vi "Switching Passive Active, Waveform Parameters.vi"(0 "error in":errorcluster, 3 "waveform":i32=1 min=1 step=1) -> (7 "error out":errorcluster, 10 "MICS Command":string)   [LabVIEW 2010]
doc: "This function builds the Patient Stim programs for Switching Passive Active."
panel:
  in  "Patient Stim Program":string[][](table)=[["ProgramNumber", "4", "4"], ["ProgramDefined", "1", "1"], ["ProgramDisabled", "0", "0"], ["ProgramName", "4_P-A Switch_3x8", "4_P-A Switch_2x12"], ["AllowedFrequencies[0]", "0xFF", "0xFF"], ["AllowedFrequencies[1]", "0xFF", "0xFF"], ["AllowedFrequencies[2]", "0xFF", "0xFF"], ["AllowedFrequencies[3]", "0xFF", "0xFF"], ["AllowedFrequencies[4]", "0xFF", "0xFF"], ["AllowedFrequencies[5]", "0xFF", "0xFF"], ["AllowedFrequencies[6]", "0xFF", "0xFF"], ["AllowedFrequencies[7]", "0xFF", "0xFF"], ["ProgramFrequencyIndex", "21", "21"], ["DefinedPulseMap", "15", "15"], ["PulseNamePA", "P1", "P1"], ["AmplitudeLowLimitPA", "5000", "5000"], ["AmplitudeStepPA", "15", "15"], ["AmplitudeStepIndexPA", "1", "1"], ["PulseWidthLowLimitPA", "400", "400"], ["PulseWidthHighLimitPA", "600", "600"], ["PulseWidthPA", "500", "500"], ["ElectrodeAmpPercentagePA[CH01]", "0", "0"], ["ElectrodeAmpPercentagePA[CH02]", "0", "0"], ["ElectrodeAmpPercentagePA[CH03]", "0", "0"], ["ElectrodeAmpPercentagePA[CH04]", "0", "0"], ["ElectrodeAmpPercentagePA[CH05]", "0", "0"], ["ElectrodeAmpPercentagePA[CH06]", "0", "0"], ["ElectrodeAmpPercentagePA[CH07]", "0", "0"], ["ElectrodeAmpPercentagePA[CH08]", "0", "0"], ["ElectrodeAmpPercentagePA[CH09]", "0", "0"], ["ElectrodeAmpPercentagePA[CH10]", "0", "0"], ["ElectrodeAmpPercentagePA[CH11]", "0", "0"], ["ElectrodeAmpPercentagePA[CH12]", "0", "0"], ["ElectrodeAmpPercentagePA[CH13]", "0", "0"], ["ElectrodeAmpPercentagePA[CH14]", "0", "0"], ["ElectrodeAmpPercentagePA[CH15]", "0", "0"], ["ElectrodeAmpPercentagePA[CH16]", "100", "0"], ["ElectrodeAmpPercentagePA[CH17]", "-100", "100"], ["ElectrodeAmpPercentagePA[CH18]", "0", "0"], ["ElectrodeAmpPercentagePA[CH19]", "0", "-100"], ["ElectrodeAmpPercentagePA[CH20]", "0", "0"], ["ElectrodeAmpPercentagePA[CH21]", "0", "0"], ["ElectrodeAmpPercentagePA[CH22]", "0", "0"], ["ElectrodeAmpPercentagePA[CH23]", "0", "0"], ["ElectrodeAmpPercentagePA[CH24]", "0", "0"], ["ElectrodeAmpPercentagePA[CH25]", "0", "0"], ["ElectrodeAmpPercentagePA[CH26]", "0", "0"], ["PulseNamePB", "P2", "P2"], ["AmplitudeLowLimitPB", "4000", "4000"], ["AmplitudeStepPB", "15", "15"], ["AmplitudeStepIndexPB", "1", "1"], ["PulseWidthLowLimitPB", "400", "400"], ["PulseWidthHighLimitPB", "600", "600"], ["PulseWidthPB", "500", "500"], ["ElectrodeAmpPercentagePB[CH01]", "0", "0"], ["ElectrodeAmpPercentagePB[CH02]", "0", "0"], ["ElectrodeAmpPercentagePB[CH03]", "0", "0"], ["ElectrodeAmpPercentagePB[CH04]", "0", "0"], ["ElectrodeAmpPercentagePB[CH05]", "0", "0"], ["ElectrodeAmpPercentagePB[CH06]", "0", "0"], ["ElectrodeAmpPercentagePB[CH07]", "0", "0"], ["ElectrodeAmpPercentagePB[CH08]", "0", "0"], ["ElectrodeAmpPercentagePB[CH09]", "0", "0"], ["ElectrodeAmpPercentagePB[CH10]", "0", "0"], ["ElectrodeAmpPercentagePB[CH11]", "0", "0"], ["ElectrodeAmpPercentagePB[CH12]", "0", "0"], ["ElectrodeAmpPercentagePB[CH13]", "0", "0"], ["ElectrodeAmpPercentagePB[CH14]", "0", "0"], ["ElectrodeAmpPercentagePB[CH15]", "0", "0"], ["ElectrodeAmpPercentagePB[CH16]", "100", "0"], ["ElectrodeAmpPercentagePB[CH17]", "-100", "100"], ["ElectrodeAmpPercentagePB[CH18]", "0", "0"], ["ElectrodeAmpPercentagePB[CH19]", "0", "-100"], ["ElectrodeAmpPercentagePB[CH20]", "0", "0"], ["ElectrodeAmpPercentagePB[CH21]", "0", "0"], ["ElectrodeAmpPercentagePB[CH22]", "0", "0"], ["ElectrodeAmpPercentagePB[CH23]", "0", "0"], ["ElectrodeAmpPercentagePB[CH24]", "0", "0"], ["ElectrodeAmpPercentagePB[CH25]", "0", "0"], ["ElectrodeAmpPercentagePB[CH26]", "0", "0"], ["PulseNamePC", "P3", "P3"], ["AmplitudeLowLimitPC", "3000", "3000"], ["AmplitudeStepPC", "15", "15"], ["AmplitudeStepIndexPC", "1", "1"], ["PulseWidthLowLimitPC", "400", "400"], ["PulseWidthHighLimitPC", "600", "600"], ["PulseWidthPC", "500", "500"], ["ElectrodeAmpPercentagePC[CH01]", "0", "0"], ["ElectrodeAmpPercentagePC[CH02]", "0", "0"], ["ElectrodeAmpPercentagePC[CH03]", "0", "0"], ["ElectrodeAmpPercentagePC[CH04]", "0", "0"], ["ElectrodeAmpPercentagePC[CH05]", "0", "0"], ["ElectrodeAmpPercentagePC[CH06]", "0", "0"], ["ElectrodeAmpPercentagePC[CH07]", "0", "0"], ["ElectrodeAmpPercentagePC[CH08]", "0", "0"], ["ElectrodeAmpPercentagePC[CH09]", "0", "0"], ["ElectrodeAmpPercentagePC[CH10]", "0", "0"], ["ElectrodeAmpPercentagePC[CH11]", "0", "0"], ["ElectrodeAmpPercentagePC[CH12]", "0", "0"], ["ElectrodeAmpPercentagePC[CH13]", "0", "0"], ["ElectrodeAmpPercentagePC[CH14]", "0", "0"], ["ElectrodeAmpPercentagePC[CH15]", "0", "0"], ["ElectrodeAmpPercentagePC[CH16]", "100", "0"], ["ElectrodeAmpPercentagePC[CH17]", "-100", "100"], ["ElectrodeAmpPercentagePC[CH18]", "0", "0"], ["ElectrodeAmpPercentagePC[CH19]", "0", "-100"], ["ElectrodeAmpPercentagePC[CH20]", "0", "0"], ["ElectrodeAmpPercentagePC[CH21]", "0", "0"], ["ElectrodeAmpPercentagePC[CH22]", "0", "0"], ["ElectrodeAmpPercentagePC[CH23]", "0", "0"], ["ElectrodeAmpPercentagePC[CH24]", "0", "0"], ["ElectrodeAmpPercentagePC[CH25]", "0", "0"], ["ElectrodeAmpPercentagePC[CH26]", "0", "0"], ["PulseNamePD", "P4", "P4"], ["AmplitudeLowLimitPD", "2000", "2000"], ["AmplitudeStepPD", "15", "15"], ["AmplitudeStepIndexPD", "1", "1"], ["PulseWidthLowLimitPD", "400", "400"], ["PulseWidthHighLimitPD", "600", "600"], ["PulseWidthPD", "500", "500"], ["ElectrodeAmpPercentagePD[CH01]", "0", "0"], ["ElectrodeAmpPercentagePD[CH02]", "0", "0"], ["ElectrodeAmpPercentagePD[CH03]", "0", "0"], ["ElectrodeAmpPercentagePD[CH04]", "0", "0"], ["ElectrodeAmpPercentagePD[CH05]", "0", "0"], ["ElectrodeAmpPercentagePD[CH06]", "0", "0"], ["ElectrodeAmpPercentagePD[CH07]", "0", "0"], ["ElectrodeAmpPercentagePD[CH08]", "0", "0"], ["ElectrodeAmpPercentagePD[CH09]", "0", "0"], ["ElectrodeAmpPercentagePD[CH10]", "0", "0"], ["ElectrodeAmpPercentagePD[CH11]", "0", "0"], ["ElectrodeAmpPercentagePD[CH12]", "0", "0"], ["ElectrodeAmpPercentagePD[CH13]", "0", "0"], ["ElectrodeAmpPercentagePD[CH14]", "0", "0"], ["ElectrodeAmpPercentagePD[CH15]", "0", "0"], ["ElectrodeAmpPercentagePD[CH16]", "100", "0"], ["ElectrodeAmpPercentagePD[CH17]", "-100", "100"], ["ElectrodeAmpPercentagePD[CH18]", "0", "0"], ["ElectrodeAmpPercentagePD[CH19]", "0", "-100"], ["ElectrodeAmpPercentagePD[CH20]", "0", "0"], ["ElectrodeAmpPercentagePD[CH21]", "0", "0"], ["ElectrodeAmpPercentagePD[CH22]", "0", "0"], ["ElectrodeAmpPercentagePD[CH23]", "0", "0"], ["ElectrodeAmpPercentagePD[CH24]", "0", "0"], ["ElectrodeAmpPercentagePD[CH25]", "0", "0"], ["ElectrodeAmpPercentagePD[CH26]", "0", "0"]] caption="Table 1"
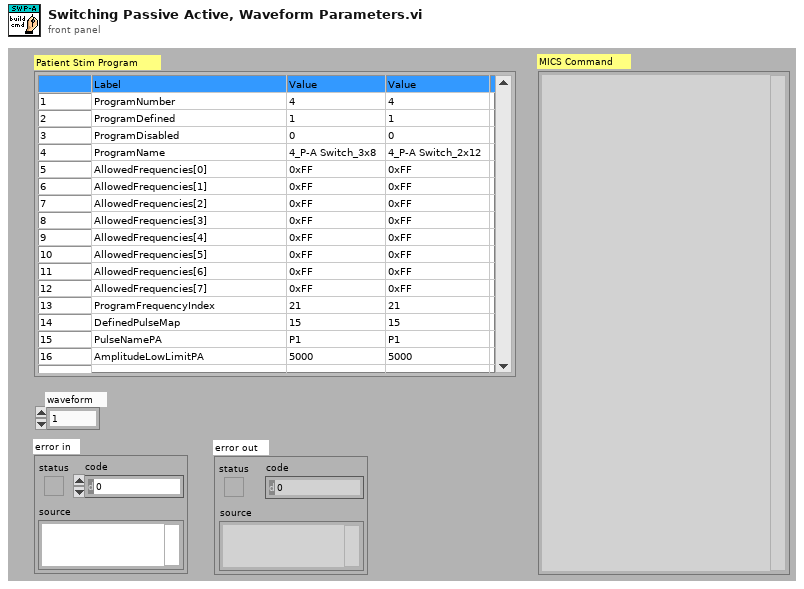
[diagram p1: front panel]
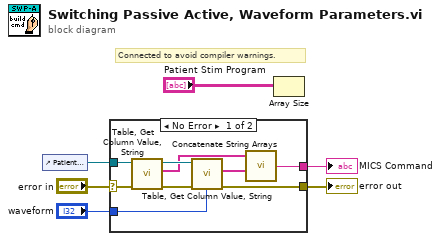
[diagram p0: block diagram]
diagram:
  # "Connected to avoid compiler warnings."
  n1 = control-ref of="Patient Stim Program"() -> (w1:refnum<vi>)
  n2 = case shown="No Error" "error in" {
    selector: "error in" -> [w15 w16]
    tunnel: w1 -> [w12 _]
    tunnel: [w13 w16] -> w6
    tunnel: "waveform" -> [w10 _]
    tunnel: [w7 _] -> w3
    frame No Error {
      n3 = call "Table, Get Column Value, String.vi"("error in"=w15, "Tbl Refnum"=w12) -> ("error out"=w14:errorcluster, "Value"=w9:string[], "Tbl Refnum out"=w11:refnum<vi>)  [unwired: 6 in]
      n4 = call "Table, Get Column Value, String.vi"("error in"=w14, "Tbl Refnum"=w11, "column (0)"=w10) -> ("error out"=w13:errorcluster, "Value"=w8:string[])  [unwired: 5 in, 1 out]
      n5 = call "Concatenate String Arrays.vi"("array1"=w9, "array2"=w8) -> ("string out"=w7:string)  [unwired: 3 in]
    }
    frame Error {
    }
  }
  "error out" <- w6
  "MICS Command" <- w3
  n6 = Array Size(array="Patient Stim Program") -> ()  [unwired: 1 out]
